vi "Qualify Device Name.vi"(8 "error in":errorcluster, 10 "Device":string, 11 "Config in":refnum<class "Config.lvclass">) -> (0 "error out":errorcluster, 2 "Illegal Name":bool, 3 "Config out":refnum<class "Config.lvclass">)   [LabVIEW 2023, in "Config.lvlib" / "Config.lvclass"]
uses:
  Config.lvclass
  Config.lvclass/Config.ctl
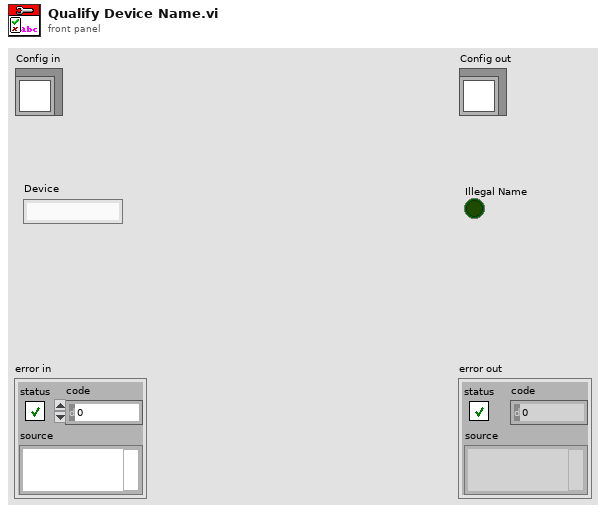
[diagram p1: front panel]
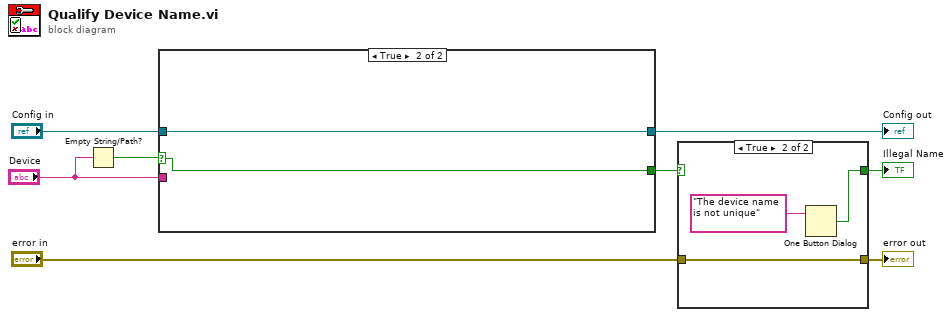
[diagram p0: block diagram]
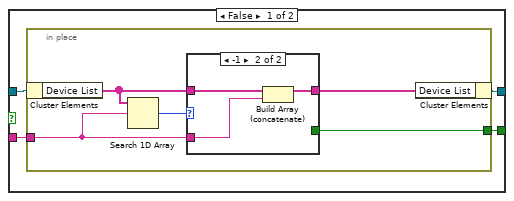
[diagram p2: hidden frame]
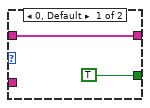
[diagram p3: hidden frame]
diagram:
  n1 = Empty String/Path?(string/path="Device") -> (empty?=w1:bool)
  n2 = case shown="True" w1 {
    selector: w1 -> [_ w24]
    tunnel: "Config in" -> [w12 w23]
    tunnel: [w11 w23] -> w7
    tunnel: "Device" -> [w10 _]
    tunnel: [w9 w24] -> w6
    frame False {
      n3 = in-place {
        in-place-border: w10 -> [w14]
        in-place-border: [w13] -> w9
        n4 = in-place-cluster #1(w12) -> ("Device List"=w16:string[])
        n5 = Search 1D Array(1D array=w16, element=w14) -> (index of element=w17:i32)  [unwired: 1 in]
        n6 = case shown="-1" w17 {
          tunnel: w16 -> [w19 w21]
          tunnel: [w19 w20] -> w15
          tunnel: w14 -> [_ w22]
          tunnel: [TRUE _] -> w13
          frame 0, Default {
          }
          frame -1 {
            n7 = Build Array (concatenate)(w21, w22) -> (w20:string[])
          }
        }
        n8 = in-place-cluster #1("Device List"=w15) -> (w11:refnum<class "Config.lvclass">)
      }
    }
    frame True {
    }
  }
  "Config out" <- w7
  n9 = case shown="True" w6 {
    selector: w6 -> [w25 _]
    tunnel: "error in" -> [w26 w28]
    tunnel: [w25 w29] -> w4
    tunnel: [w26 w28] -> w3
    frame False {
    }
    frame True {
      n10 = One Button Dialog(message="The device name is not unique") -> (true=w29:bool)  [unwired: 1 in]
    }
  }
  "error out" <- w3
  "Illegal Name" <- w4
